vi "Compare New Plot and Sum X Arrays.vi"(5 "Different Y Scale":bool, 6 "epsilon (machine)":dbl=2.220446049250313e-16, 7 "Different X Scale":bool, 8 "Existing Y Array":dbl[](array[numeric]), 9 "New X Array in":dbl[](array[numeric]), 10 "Different X Axis":bool, 11 "Existing X Array":dbl[](array[numeric])) -> (0 "Y Array out":dbl[](array[numeric]), 1 "Cancel":bool, 2 "Keep Plot":bool, 3 "X Array out":dbl[](array[numeric]))   [LabVIEW 2019]
uses:
  Axis Differences.ctl
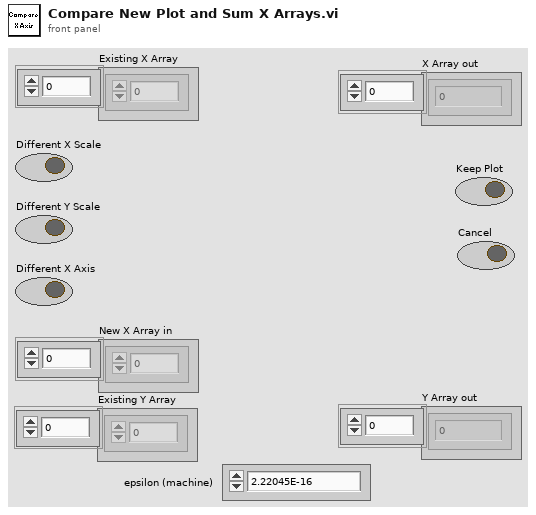
[diagram p1: front panel]
types:
  T1 = typedef "Axis Differences.ctl" = enum16{"Different X Scale", "Different Y Scale", "Different X Axis"}
  T2 = enum16{"Left Button", "Center Button", "Right Button", "Window Close"}
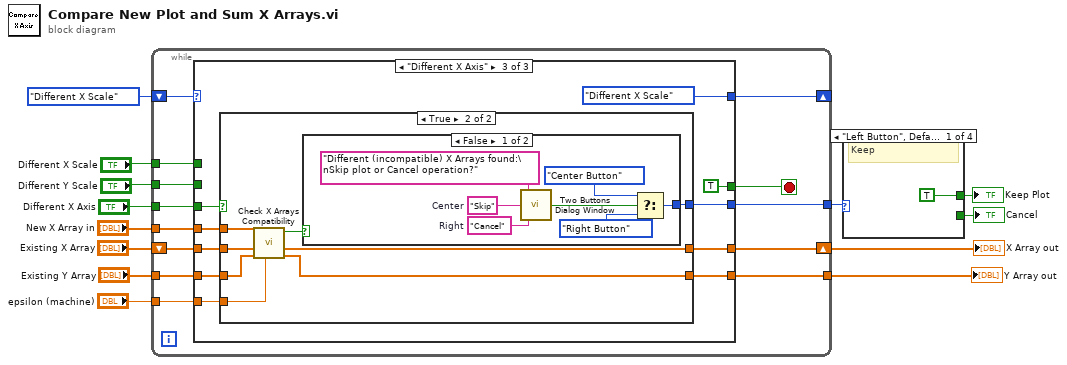
[diagram p0: block diagram]
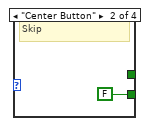
[diagram p2: hidden frame]
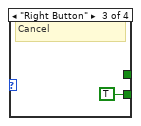
[diagram p3: hidden frame]
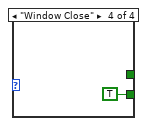
[diagram p4: hidden frame]
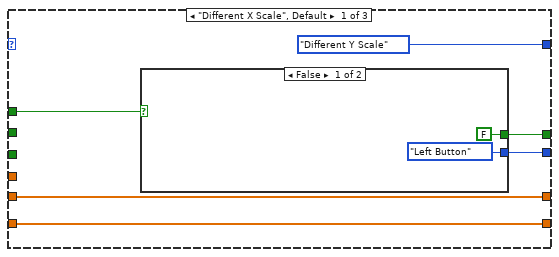
[diagram p5: hidden frame]
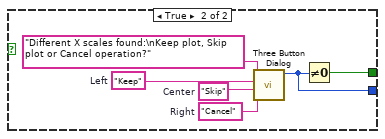
[diagram p6: hidden frame]
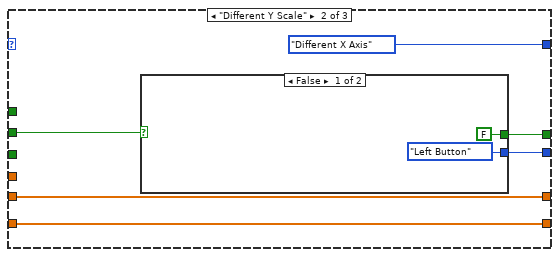
[diagram p7: hidden frame]
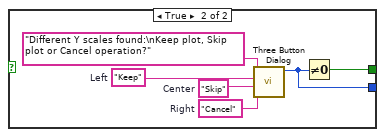
[diagram p8: hidden frame]
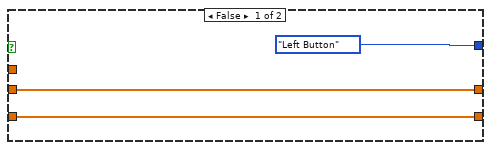
[diagram p9: hidden frame]
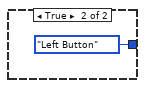
[diagram p10: hidden frame]
diagram:
  n1 = while {
    shift-right: [w25] -> _
    shift-left: Axis_Differences."Different X Scale" -> [w26]
    tunnel: [w23] -> w12
    tunnel: "Different X Scale" -> [w22]
    tunnel: "Different Y Scale" -> [w21]
    tunnel: "Different X Axis" -> [w20]
    shift-right: [w18] -> w5
    shift-left: "Existing X Array" -> [w19]
    tunnel: "New X Array in" -> [w17]
    tunnel: "Existing Y Array" -> [w16]
    tunnel: [w15] -> w2
    tunnel: "epsilon (machine)" -> [w14]
    stop <- w24 stop-if-true
    n2 = case shown="\"Different X Axis\"" w26 {
      tunnel: [Axis_Differences."Different Y Scale" Axis_Differences."Different X Axis" Axis_Differences."Different X Scale"] -> w25
      tunnel: [w31 w45 TRUE] -> w24
      tunnel: [w30 w44 w63] -> w23
      tunnel: w22 -> [w29 _ _]
      tunnel: w21 -> [_ w43 _]
      tunnel: w20 -> [_ _ w61]
      tunnel: w19 -> [w28 w42 w60]
      tunnel: [w28 w42 w59] -> w18
      tunnel: w17 -> [_ _ w58]
      tunnel: w16 -> [w27 w41 w57]
      tunnel: [w27 w41 w56] -> w15
      tunnel: w14 -> [_ _ w55]
      frame "Different X Scale", Default {
        n3 = case shown="False" w29 {
          tunnel: [FALSE w36] -> w31
          tunnel: [T2."Left Button" ("Which Button?") w35] -> w30
          frame False {
          }
          frame True {
            w37 = "Cancel"  # Right
            w38 = "Keep"  # Left
            w39 = "Skip"  # Center
            n4 = call <vilib>:"Three Button Dialog.vi"("Right Button Text (\"Cancel\")"=w37, "Center Button Text (\"No\")"=w39, "Left Button Text (\"Yes\")"=w38, "message"="Different X scales found:\nKeep plot, Skip plot or Cancel operation?") -> ("Which Button?"=w35:T2)  [unwired: 7 in]
            n5 = Not Equal To 0?(x=w35) -> (x != 0?=w36:bool)
          }
        }
      }
      frame "Different Y Scale" {
        n6 = case shown="False" w43 {
          tunnel: [FALSE w50] -> w45
          tunnel: [T2."Left Button" ("Which Button?") w49] -> w44
          frame False {
          }
          frame True {
            w51 = "Cancel"  # Right
            w52 = "Keep"  # Left
            w53 = "Skip"  # Center
            n7 = call <vilib>:"Three Button Dialog.vi"("Right Button Text (\"Cancel\")"=w51, "Center Button Text (\"No\")"=w53, "Left Button Text (\"Yes\")"=w52, "message"="Different Y scales found:\nKeep plot, Skip plot or Cancel operation?") -> ("Which Button?"=w49:T2)  [unwired: 7 in]
            n8 = Not Equal To 0?(x=w49) -> (x != 0?=w50:bool)
          }
        }
      }
      frame "Different X Axis" {
        n9 = case shown="True" w61 {
          tunnel: [T2."Left Button" ("Which Button?") w75] -> w63
          tunnel: w60 -> [w66 w72]
          tunnel: [w66 w71] -> w59
          tunnel: w58 -> [_ w74]
          tunnel: w57 -> [w65 w70]
          tunnel: [w65 w69] -> w56
          tunnel: w55 -> [_ w68]
          frame False {
          }
          frame True {
            n10 = call "Check X Arrays Compatibility.vi"("epsilon (machine)"=w68, "Existing Y Array"=w70, "Existing X Array in"=w72, "New X Array in"=w74) -> ("Y Array out"=w69:dbl[], "X Array out"=w71:dbl[], "Compatible Arrays?"=w73:bool)  [unwired: 5 in]
            n11 = case shown="False" w73 {
              tunnel: [w76 T2."Left Button" ("Which Button?")] -> w75
              frame False {
                w81 = "Cancel"  # Right
                w82 = "Skip"  # Center
                n12 = call "Two Buttons Dialog Window.vi"("Cancel Button Text"=w81, "OK Button Text"=w82, "Message"="Different (incompatible) X Arrays found:\nSkip plot or Cancel operation?" ("message")) -> ("OK?"=w79:bool)
                n13 = Select(t=T2."Center Button" ("Which Button?"), s=w79, f=T2."Right Button" ("Which Button?")) -> (s? t:f=w76:T2)
              }
              frame True {
              }
            }
          }
        }
      }
    }
  }
  "X Array out" <- w5
  "Y Array out" <- w2
  n14 = case shown="\"Left Button\", Default" w12 {
    tunnel: [TRUE ("Keep Plot") _ _ _] -> w11
    tunnel: [_ FALSE ("Cancel") TRUE ("Cancel") TRUE ("Cancel")] -> w10
    frame "Left Button", Default {
      # "Keep"
    }
    frame "Center Button" {
      # "Skip"
    }
    frame "Right Button" {
      # "Cancel"
    }
    frame "Window Close" {
    }
  }
  "Keep Plot" <- w11
  "Cancel" <- w10
